vi "Activate License Local.vi"() -> ()   [LabVIEW 2018]
doc: "Demonstrates how to activate a license through using local license file. (The license file is usually provided"
panel:
  out "result":i8
  in  "Product":string
  in  "license file":path
  # "Overview: Demonstrates how to activate a license through using local license file. (The license file is usually provided by the manufacturer of this software.\nRequirements: Windows.\nInstructions: \n1. Fill in the product name (opencv_dnn, openvino, onnx_gpu, tensorRT and etc), License file in the controls.\n2. Run the VI.\n3. When the software is successfully activated, the VI returns 1, otherwise it is 0"
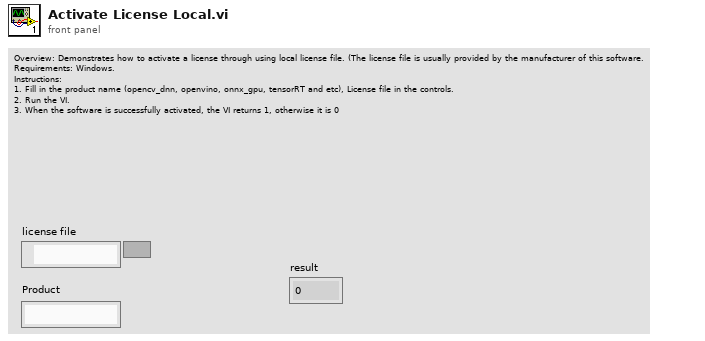
[diagram p1: front panel]
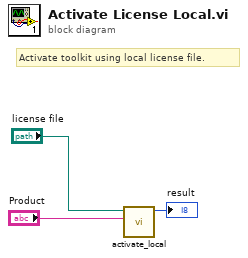
[diagram p0: block diagram]
diagram:
  # "Activate toolkit using local license file."
  n1 = call "activate_local.vi"("Product Name"="Product", "license file"="license file") -> ("result"=→"result":i8)  [unwired: 8 in, 1 out]
